vi "Ch_data_pattern_8_save (SubVI).vi"(7 "error in":errorcluster, 14 "T Cluster":T1, 15 "Activate!":bool, 17 "file":refnum<file>) -> (27 "error out":errorcluster)   [LabVIEW 2015]
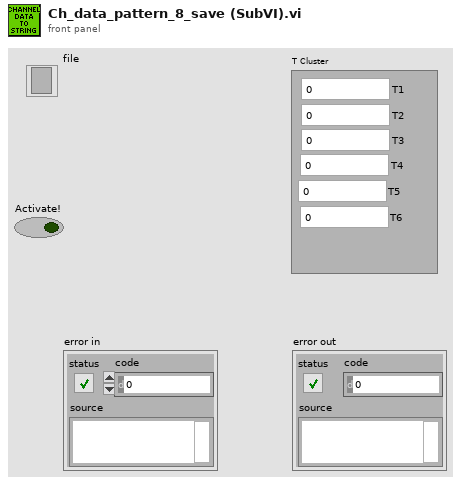
[diagram p1: front panel]
types:
  T1 = cluster{"T1":dbl, "T2":dbl, "T3":dbl, "T4":dbl, "T5":dbl, "T6":dbl}
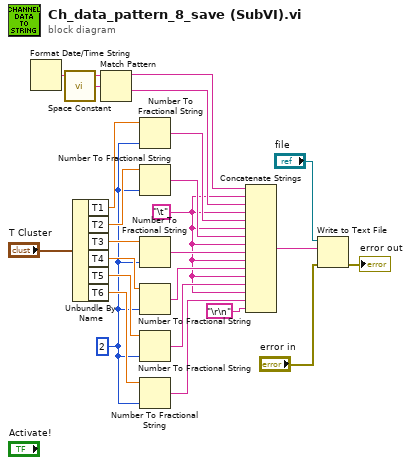
[diagram p0: block diagram]
diagram:
  w1 = i16 2 ("precision (6)")
  w4 = "\t"
  n1 = Format Date/Time String() -> (date/time string=w22:string)  [unwired: 3 out]
  n2 = call <vilib>:"Space Constant.vi"() -> ("String"=w23:string)
  n3 = Unbundle By Name("T Cluster") -> ("T1"=w19:dbl, "T2"=w20:dbl, "T3"=w9:dbl, "T4"=w8:dbl, "T5"=w7:dbl, "T6"=w5:dbl)
  n4 = Match Pattern(string=w22, regular expression=w23) -> (before substring=w12:string, after substring=w11:string)  [unwired: 3 out]
  n5 = Number To Fractional String(number=w19, precision (6)=w1) -> (F-format string=w18:string)  [unwired: 2 out]
  n6 = Number To Fractional String(number=w20, precision (6)=w1) -> (F-format string=w14:string)  [unwired: 2 out]
  n7 = Number To Fractional String(number=w9, precision (6)=w1) -> (F-format string=w17:string)  [unwired: 2 out]
  n8 = Number To Fractional String(number=w8, precision (6)=w1) -> (F-format string=w16:string)  [unwired: 2 out]
  n9 = Number To Fractional String(number=w7, precision (6)=w1) -> (F-format string=w6:string)  [unwired: 2 out]
  n10 = Number To Fractional String(number=w5, precision (6)=w1) -> (F-format string=w3:string)  [unwired: 2 out]
  n11 = Concatenate Strings(w12, w4, w11, w4, w18, w4, w14, w4, w17, w4, w16, w4, w6, w4, w3, "\r\n") -> (w10:string)
  n12 = Write to Text File(file (use dialog)="file", text=w10, error in="error in") -> (error out=→"error out":errorcluster)  [unwired: 3 out]
